vi "CRYGet Selected Data in Legend.vi"(10 "Right Clicked Row":i32=-1, 11 "Legend Ref":refnum<vi>) -> (3 "Selected Rows":i32[](array[numeric]))   [LabVIEW 2013]
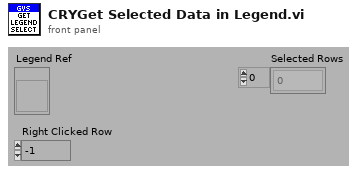
[diagram p1: front panel]
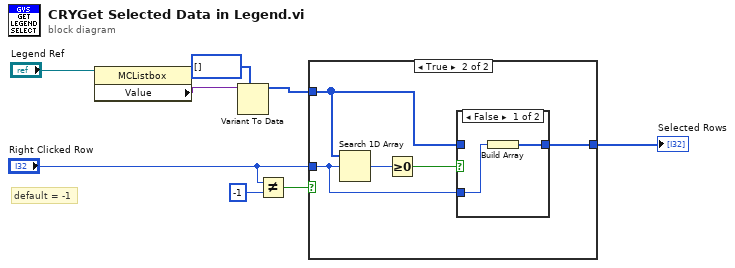
[diagram p0: block diagram]
diagram:
  # "default = -1"
  n1 = property class="MCListbox"(reference="Legend Ref") -> ("Value"=w5:variant)  [unwired: 1 in, 2 out]
  n2 = Variant To Data(type=i32[] [] ("Rows"), Variant=w5) -> (data=w4:i32[])  [unwired: 1 in, 1 out]
  n3 = Not Equal?(x="Right Clicked Row", y=-1) -> (x != y?=w2:bool)
  n4 = case shown="True" w2 {
    tunnel: [w9 w13] -> w8
    tunnel: w4 -> [w9 w12]
    tunnel: "Right Clicked Row" -> [_ w10]
    frame False {
    }
    frame True {
      n5 = Search 1D Array(1D array=w12, element=w10) -> (index of element=w14:i32)  [unwired: 1 out]
      n6 = Greater Or Equal To 0?(x=w14) -> (x >= 0?=w11:bool)
      n7 = case shown="False" w11 {
        tunnel: [w15 w17] -> w13
        tunnel: w12 -> [_ w17]
        tunnel: w10 -> [w16 _]
        frame False {
          n8 = Build Array(w16) -> (w15:i32[])
        }
        frame True {
        }
      }
    }
  }
  "Selected Rows" <- w8
